vi "Three-ENC.vi"(7 "Reset":bool[](array[boolean]), 8 "Error In":errorcluster) -> (0 "Error Out":errorcluster, 3 "Counter Value":dbl[](array[numeric]) format="%.2f")   [LabVIEW 2019]
uses:
  <vilib>/Utility/error.llb/Error Cluster From Error Code.vi
  <vilib>/myRIO/Common/Instrument Driver Framework/myRIO v1.0/Encoder/vis/myRIO v1.0 Read Encoder.vi
  <vilib>/myRIO/Instrument Drivers/Onboard IO/Encoder/Encoder.lvlib
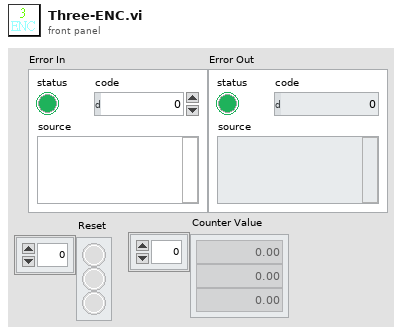
[diagram p1: front panel]
types:
  T1 = cluster{"馬達PWM腳位":tag, "馬達DIR腳位":tag[], "馬達Encoder角位":tag}[]
  T2 = cluster{"馬達PWM腳位":tag, "馬達DIR腳位":tag[], "馬達Encoder角位":tag}
  T3 = typedef "Encoder.lvlib/Encoder Reference.ctl" = cluster{"myRIO Reference":T4, "Encoder Channels Enum":T8}
  T4 = typedef "myRIO Generic Hardware Reference.ctl" = cluster{"myRIO Model":T5, "myRIO Hardware Reference":T6}
  T5 = typedef "Hardware Version Enum.ctl" = enum16{"Unknown", "myRIO-1900", "myRIO-1950", "roboRIO", "NI ELVIS RIO CM", "ELVIS III"}
  T6 = typedef "myRIO v1.0 Reference.ctl" = cluster{"Generic FPGA Reference":T7, "Allow multiple opens":bool}
  T7 = typedef "Generic FPGA Reference.ctl" = refnum<k20>
  T8 = typedef "Encoder Channels Enum.ctl" = enum16{"Not Connected", "C/ENC0", "C/ENC1", "A/ENC", "A/ENC0", "A/ENC1", "A/ENC2", "A/ENC3", "A/ENC4", "A/ENC5", "A/ENC6", "A/ENC7", "A/ENC8", "A/ENC9", "B/ENC", "B/ENC0", "B/ENC1", "B/ENC2", "B/ENC3", "B/ENC4", "B/ENC5", "B/ENC6", "B/ENC7", "B/ENC8", "B/ENC9", "DIO/ENC0", "DIO/ENC1", "DIO/ENC2", "DIO/ENC3", "DIO/ENC4"}
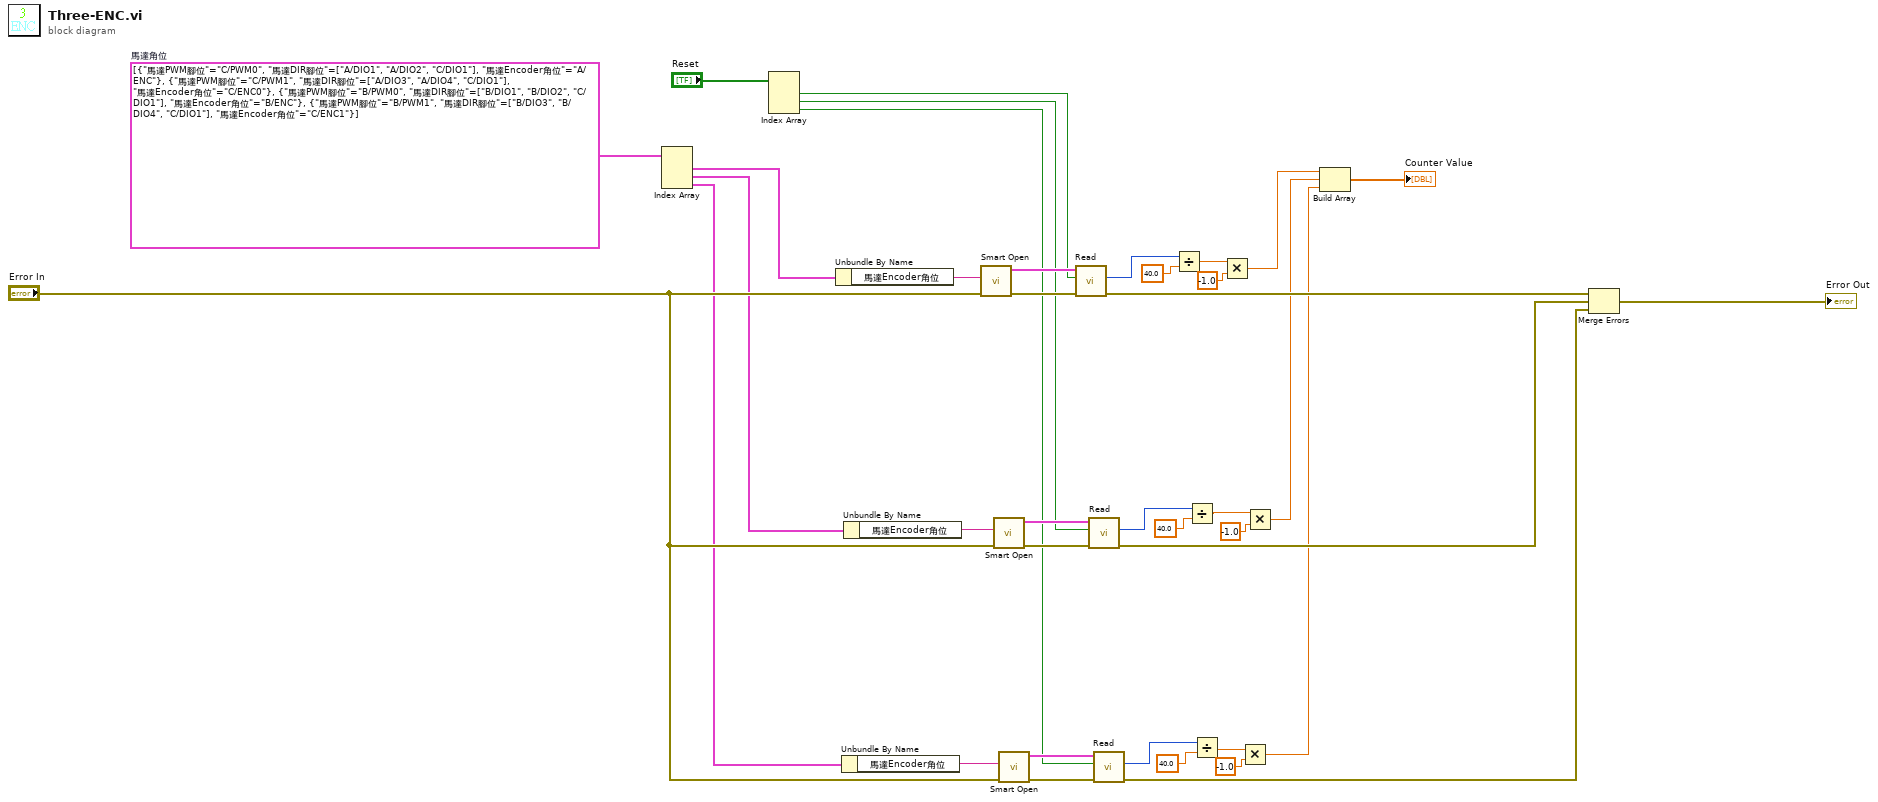
[diagram p0: block diagram]
diagram:
  w33 = T1 [{"馬達PWM腳位"="C/PWM0", "馬達DIR腳位"=["A/DIO1", "A/DIO2", "C/DIO1"], "馬達Encoder角位"="A/ENC"}, {"馬達PWM腳位"="C/PWM1", "馬達DIR腳位"=["A/DIO3", "A/DIO4", "C/DIO1"], "馬達Encoder角位"="C/ENC0"}, {"馬達PWM腳位"="B/PWM0", "馬達DIR腳位"=["B/DIO1", "B/DIO2", "C/DIO1"], "馬達Encoder角位"="B/ENC"}, {"馬達PWM腳位"="B/PWM1", "馬達DIR腳位"=["B/DIO3", "B/DIO4", "C/DIO1"], "馬達Encoder角位"="C/ENC1"}]  # 馬達角位
  n1 = Index Array(array=w33) -> (element #1=w6:T2, element #2=w4:T2, element #3=w3:T2)  [unwired: 3 in]
  n2 = Index Array(array="Reset") -> (element #1=w23:bool, element #2=w22:bool, element #3=w21:bool)  [unwired: 3 in]
  n3 = Unbundle By Name(w6) -> ("馬達Encoder角位"=w5:tag)
  n4 = Unbundle By Name(w3) -> ("馬達Encoder角位"=w1:tag)
  n5 = Unbundle By Name(w4) -> ("馬達Encoder角位"=w2:tag)
  n6 = call <vilib>:"Smart Open.vi"("error in (no error)"="Error In", "Channel Name"=w5) -> ("error out"=w31:errorcluster, "Encoder Ref Out"=w32:T3)  [unwired: 8 in]
  n7 = call <vilib>:"Smart Open.vi"("error in (no error)"="Error In", "Channel Name"=w2) -> ("error out"=w28:errorcluster, "Encoder Ref Out"=w27:T3)  [unwired: 8 in]
  n8 = call <vilib>:"Smart Open.vi"("error in (no error)"="Error In", "Channel Name"=w1) -> ("error out"=w25:errorcluster, "Encoder Ref Out"=w26:T3)  [unwired: 8 in]
  n9 = call <vilib>:"Read.vi"("error in (no error)"=w31, "Reset Counter"=w23, "Encoder Ref In"=w32) -> ("error out"=w38:errorcluster, "Counter Value"=w30:i32)  [unwired: 4 in, 3 out]
  n10 = call <vilib>:"Read.vi"("error in (no error)"=w28, "Reset Counter"=w22, "Encoder Ref In"=w27) -> ("error out"=w37:errorcluster, "Counter Value"=w29:i32)  [unwired: 4 in, 3 out]
  n11 = call <vilib>:"Read.vi"("error in (no error)"=w25, "Reset Counter"=w21, "Encoder Ref In"=w26) -> ("error out"=w36:errorcluster, "Counter Value"=w24:i32)  [unwired: 4 in, 3 out]
  n12 = Divide(x=w30, y=40.0) -> (x/y=w15:dbl)
  n13 = Divide(x=w29, y=40.0) -> (x/y=w14:dbl)
  n14 = Divide(x=w24, y=40.0) -> (x/y=w12:dbl)
  n15 = Multiply(x=w15, y=-1.0) -> (x*y=w9:dbl)
  n16 = Multiply(x=w12, y=-1.0) -> (x*y=w7:dbl)
  n17 = Multiply(x=w14, y=-1.0) -> (x*y=w8:dbl)
  n18 = Build Array(w9, w8, w7) -> (→"Counter Value":dbl[])
  n19 = Merge Errors(w38, w37, w36) -> (→"Error Out":errorcluster)
